vi "SerialRPC _delete.vi"(8 "error in (no error)":errorcluster, 11 "mbed_LVLibrary.lvlib:mbed.lvclass":refnum<class "mbed.lvclass">) -> (0 "error out":errorcluster)   [LabVIEW 2011, in "mbed_LVLibrary.lvlib" / "SerialRPC.lvclass"]
doc: "This VI closes the serial port. Execute it after you have finished controlling the mbed. Just connect it to the mbed class wire that is output from mbedSerial."
uses:
  SerialRPC.lvclass
  mbed/mbed.lvclass
  SerialRPC.lvclass/SerialRPC.ctl
panel:
  in  "mbed_LVLibrary.lvlib:SerialRPC.lvclass":refnum<class "SerialRPC.lvclass">
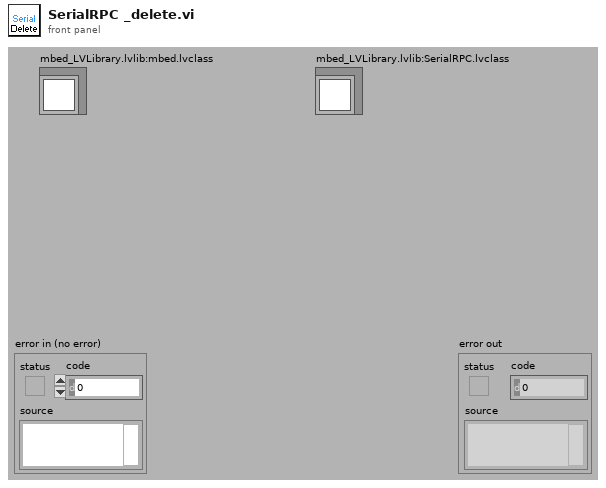
[diagram p1: front panel]
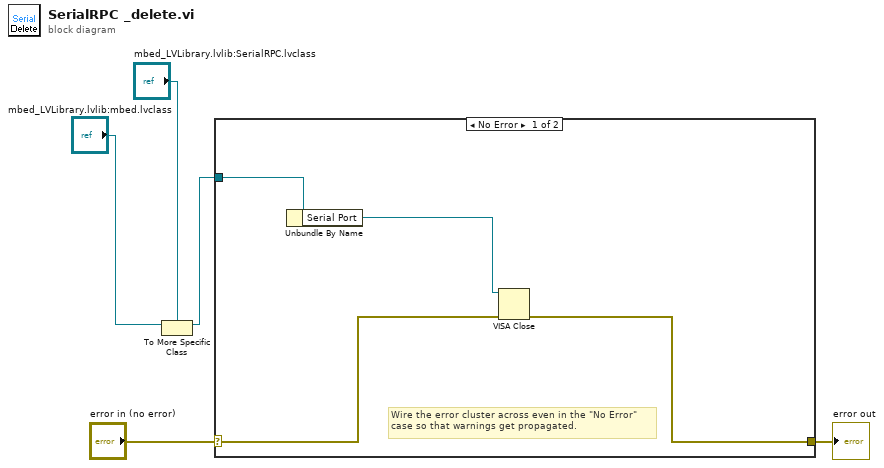
[diagram p0: block diagram]
diagram:
  n1 = To More Specific Class(target class="mbed_LVLibrary.lvlib:SerialRPC.lvclass", reference="mbed_LVLibrary.lvlib:mbed.lvclass") -> (specific class reference=w2:refnum<class "SerialRPC.lvclass">)  [unwired: 1 in, 1 out]
  n2 = case shown="No Error" "error in (no error)" {
    selector: "error in (no error)" -> [w7 w10]
    tunnel: [w6 w10] -> w4
    tunnel: w2 -> [w8 _]
    frame No Error {
      # "Wire the error cluster across even in the \"No Error\"\ncase so that warnings get propagated."
      n3 = Unbundle By Name(w8) -> ("Serial Port"=w9:refnum<visa-resource-name>)
      n4 = VISA Close(VISA resource name=w9, error in (no error)=w7) -> (error out=w6:errorcluster)
    }
    frame Error {
    }
  }
  "error out" <- w4
